vi "BuildStepListFromSteps.vi"(0 "Steps":T2(array[cluster]), 5 "Control Channels":string[](array[string]), 7 "Feedback Channels":string[](array[string]), 9 "AI":string[](array[string])) -> (4 "Step List":string[](array[string]))   [LabVIEW 2015]
panel:
  in  "Step":T1
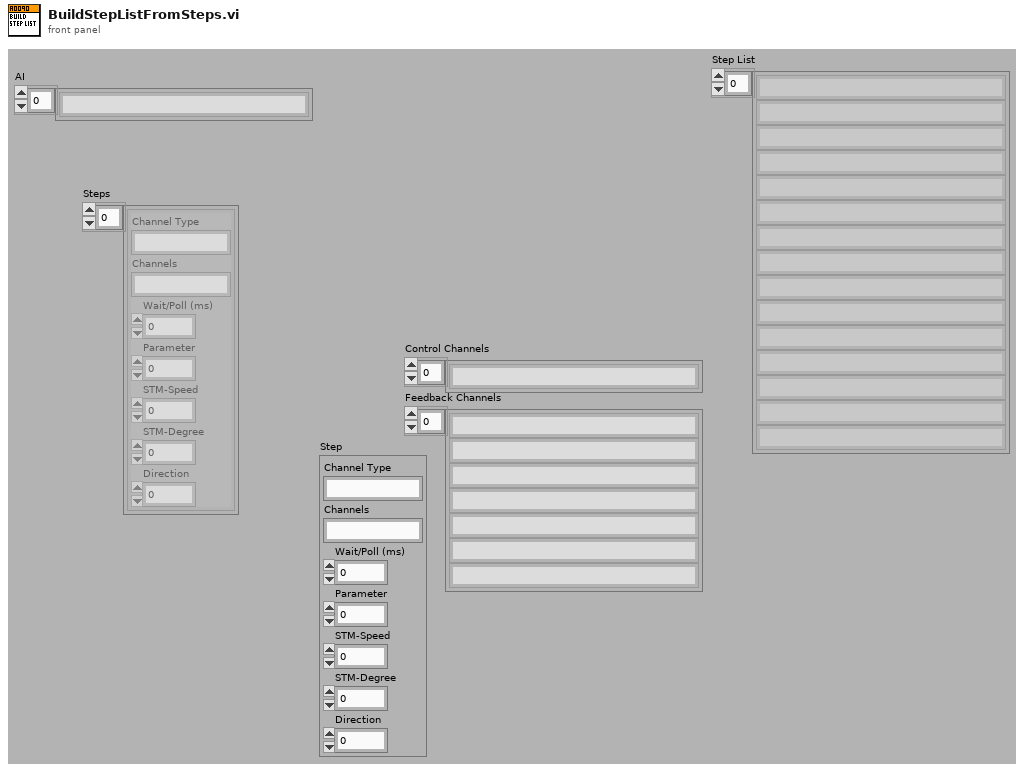
[diagram p1: front panel]
types:
  T1 = cluster{"Channel Type":string, "Channels":string, "Wait/Poll (ms)":u32, "Parameter":u8, "STM-Speed":u8, "STM-Degree":u32, "Direction":u8}
  T2 = cluster{"Channel Type":string, "Channels":string, "Wait/Poll (ms)":u32, "Parameter":u8, "STM-Speed":i32, "STM-Degree":u32, "Direction":u8}[]
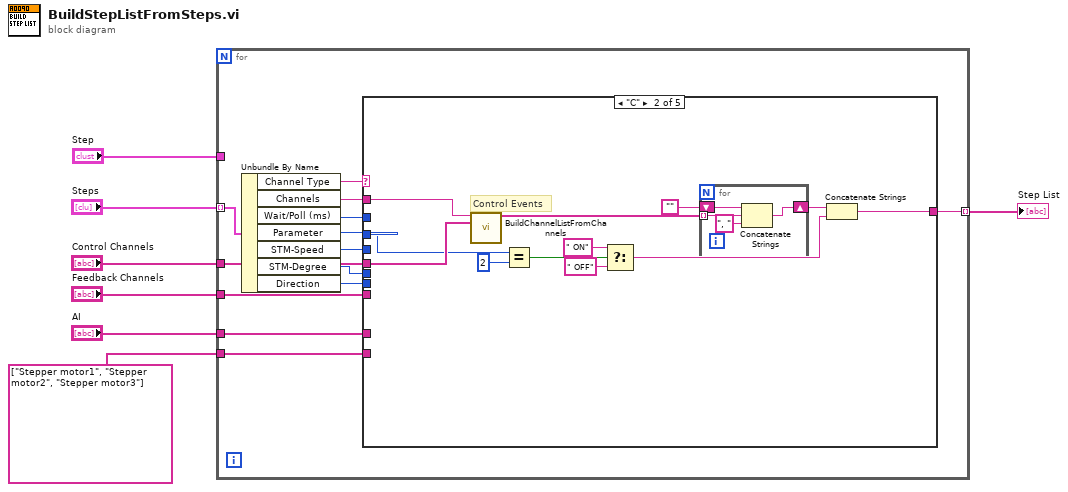
[diagram p0: block diagram]
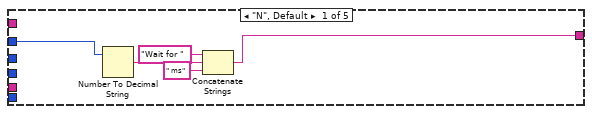
[diagram p2: hidden frame]
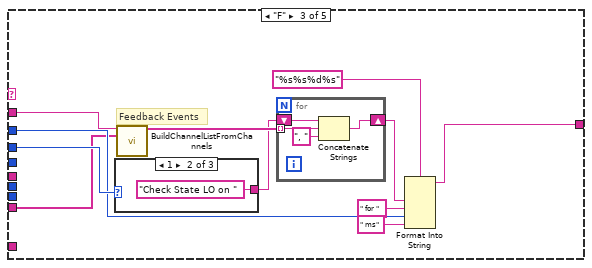
[diagram p3: hidden frame]
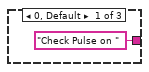
[diagram p4: hidden frame]
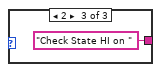
[diagram p5: hidden frame]
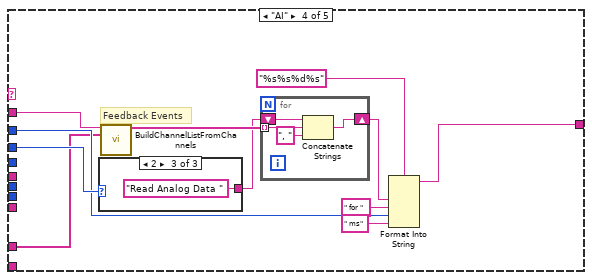
[diagram p6: hidden frame]
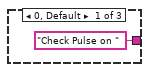
[diagram p7: hidden frame]
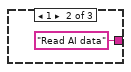
[diagram p8: hidden frame]
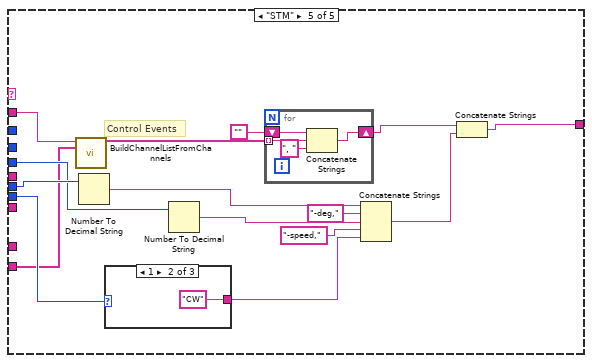
[diagram p9: hidden frame]
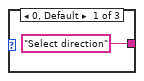
[diagram p10: hidden frame]
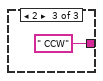
[diagram p11: hidden frame]
diagram:
  n1 = for {
    tunnel: "Steps" -> [w20] mode=indexing
    tunnel: "Control Channels" -> [w16]
    tunnel: "Feedback Channels" -> [w14]
    tunnel: [w13] -> w4 mode=indexing
    tunnel: "Step" -> [_]
    tunnel: "AI" -> [w12]
    tunnel: string[] ["Stepper motor1", "Stepper motor2", "Stepper motor3"] ("Control Channels 2") -> [w8]
    n2 = Unbundle By Name(w20) -> ("Channel Type"=w19:string, "Channels"=w17:string, "Wait/Poll (ms)"=w18:u32, "Parameter"=w15:u8, "STM-Speed"=w9:i32, "STM-Degree"=w10:u32, "Direction"=w11:u8)
    n3 = case shown="\"C\"" w19 {
      tunnel: w18 -> [w22 _ w47 w63 _]
      tunnel: w17 -> [_ w37 w52 w62 w78]
      tunnel: w16 -> [_ w36 _ _ _]
      tunnel: w15 -> [_ w31 w48 w64 _]
      tunnel: w14 -> [_ _ w46 _ _]
      tunnel: [w21 w26 w43 w61 w88] -> w13
      tunnel: w12 -> [_ _ _ w60 _]
      tunnel: w11 -> [_ _ _ _ w89]
      tunnel: w10 -> [_ _ _ _ w87]
      tunnel: w9 -> [_ _ _ _ w84]
      tunnel: w8 -> [_ _ _ _ w79]
      frame "N", Default {
        n4 = Number To Decimal String(number=w22) -> (decimal integer string=w23:string)  [unwired: 1 in]
        n5 = Concatenate Strings("Wait for ", w23, " ms" ("string")) -> (w21:string)
      }
      frame "C" {
        # "Control Events"
        n6 = call "BuildChannelListFromChannels.vi"("Channels (A:B:C:D...) (In)"=w37, "Channel Names (In)"=w36) -> ("Channel List (Out)"=w30:string[])  [unwired: 12 in, 1 out]
        n7 = Equal?(x=w31, y=u8 2) -> (x = y?=w34:bool)
        n8 = Select(t=" ON", s=w34, f=" OFF") -> (s? t:f=w28:string)
        n9 = for {
          tunnel: w30 -> [w41] mode=indexing
          shift-right: [w38] -> w27
          shift-left: "" -> [w39]
          n10 = Concatenate Strings(w39, w41, ", " ("string")) -> (w38:string)
        }
        n11 = Concatenate Strings(w27, w28) -> (w26:string)
      }
      frame "F" {
        # "Feedback Events"
        n12 = case shown="1" w48 {
          tunnel: ["Check Pulse on " "Check State LO on " "Check State HI on "] -> w42
          frame 0, Default {
          }
          frame 1 {
          }
          frame 2 {
          }
        }
        n13 = call "BuildChannelListFromChannels.vi"("Channels (A:B:C:D...) (In)"=w52, "Channel Names (In)"=w46) -> ("Channel List (Out)"=w51:string[])  [unwired: 12 in, 1 out]
        n14 = for {
          tunnel: w51 -> [w59] mode=indexing
          shift-right: [w56] -> w44
          shift-left: w42 -> [w57]
          n15 = Concatenate Strings(w57, w59, ", " ("string")) -> (w56:string)
        }
        n16 = Format Into String(format string="%s%s%d%s", w44, " for " ("input 1"), w47, " ms" ("input 3")) -> (resulting string=w43:string)  [unwired: 2 in, 1 out]
      }
      frame "AI" {
        # "Feedback Events"
        n17 = case shown="2" w64 {
          tunnel: ["Check Pulse on " "Read AI data" "Read Analog Data "] -> w65
          frame 0, Default {
          }
          frame 1 {
          }
          frame 2 {
          }
        }
        n18 = call "BuildChannelListFromChannels.vi"("Channels (A:B:C:D...) (In)"=w62, "Channel Names (In)"=w60) -> ("Channel List (Out)"=w70:string[])  [unwired: 12 in, 1 out]
        n19 = for {
          tunnel: w70 -> [w77] mode=indexing
          shift-right: [w74] -> w66
          shift-left: w65 -> [w75]
          n20 = Concatenate Strings(w75, w77, ", " ("string")) -> (w74:string)
        }
        n21 = Format Into String(format string="%s%s%d%s", w66, " for " ("input 1"), w63, " ms" ("input 3")) -> (resulting string=w61:string)  [unwired: 2 in, 1 out]
      }
      frame "STM" {
        # "Control Events"
        n22 = call "BuildChannelListFromChannels.vi"("Channels (A:B:C:D...) (In)"=w78, "Channel Names (In)"=w79) -> ("Channel List (Out)"=w92:string[])  [unwired: 12 in, 1 out]
        n23 = Number To Decimal String(number=w87) -> (decimal integer string=w86:string)  [unwired: 1 in]
        n24 = case shown="1" w89 {
          tunnel: ["Select direction" "CW" " CCW"] -> w81
          frame 0, Default {
          }
          frame 1 {
          }
          frame 2 {
          }
        }
        n25 = Number To Decimal String(number=w84) -> (decimal integer string=w83:string)  [unwired: 1 in]
        n26 = for {
          tunnel: w92 -> [w99] mode=indexing
          shift-right: [w96] -> w90
          shift-left: "" -> [w97]
          n27 = Concatenate Strings(w97, w99, ", " ("string")) -> (w96:string)
        }
        n28 = Concatenate Strings(w86, "-deg," ("string"), w83, "-speed," ("string"), w81) -> (w80:string)
        n29 = Concatenate Strings(w90, w80) -> (w88:string)
      }
    }
  }
  "Step List" <- w4
